vi "SCLN_GlobalTCPIP_Id.vi"(2 "TCPIP_Id Write":refnum<k5>, 3 "Element":i32 min=0 max=49, 4 "Operation":i32 min=0 max=1, 5 "Number of elements":i32=1 min=1 max=50) -> (0 "TCP_Id Array Out":refnum<k5>[](array[refnum]), 1 "TCPIP_Id Read":refnum<k5>)   [LabVIEW 2015]
doc: "Handle TCPIP_Id Globals Stlyle II\nThe globals are maintained in an uninitialized\nshift register, as an array of Id's.\nIt is mandatory to initialize the array to\nthe number of Id's it will contain. This is \ndone on the first invocation.\n\nINPUTS:\n Operation: 1 = WRITE, 0 = READ\n Element: Element of the array to write or read\n TCPIP_Id Write: Id to store\n\nOUTPUTS:\n TCPIP_Id Read: Id value retrieved\n TCP_Id Array Out: The entire array of Id's"
panel:
  # "1 = Write"
  # "0 = Read"
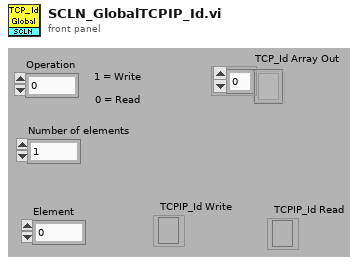
[diagram p1: front panel]
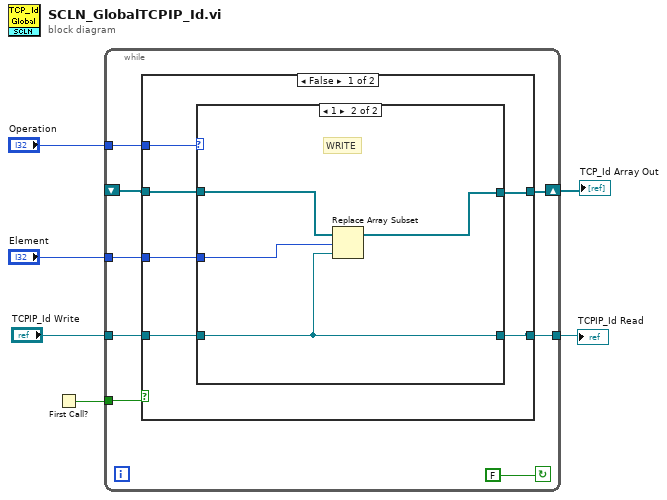
[diagram p0: block diagram]
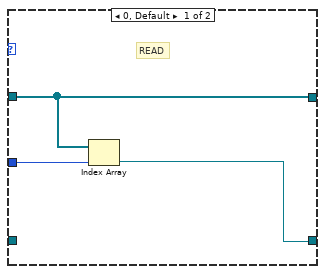
[diagram p2: hidden frame]
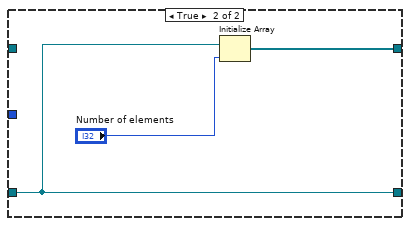
[diagram p3: hidden frame]
diagram:
  n1 = First Call?() -> (First Call?: T/F=w6:bool)
  n2 = while {
    tunnel: w6 -> [w13]
    tunnel: "Operation" -> [w12]
    tunnel: "Element" -> [w11]
    tunnel: "TCPIP_Id Write" -> [w10]
    shift-right: [w9] -> w1
    shift-left: _ -> [w7]
    tunnel: [w8] -> w2
    stop <- FALSE continue-if-true
    n3 = case shown="False" w13 {
      tunnel: w12 -> [w20 _]
      tunnel: w11 -> [w18 _]
      tunnel: w10 -> [w17 w28]
      tunnel: [w15 w29] -> w9
      tunnel: [w16 w28] -> w8
      tunnel: w7 -> [w19 _]
      frame False {
        n4 = case shown="1" w20 {
          tunnel: w19 -> [w22 w27]
          tunnel: w18 -> [w23 w26]
          tunnel: w17 -> [_ w25]
          tunnel: [w21 w25] -> w16
          tunnel: [w22 w24] -> w15
          frame 0, Default {
            # "READ"
            n5 = Index Array(array=w22, index=w23) -> (element=w21:refnum<k5>)
          }
          frame 1 {
            # "WRITE"
            n6 = Replace Array Subset(array=w27, new element=w25, index=w26) -> (w24:refnum<k5>[])
          }
        }
      }
      frame True {
        n7 = Initialize Array(w28, "Number of elements") -> (w29:refnum<k5>[])
      }
    }
  }
  "TCP_Id Array Out" <- w1
  "TCPIP_Id Read" <- w2
